vi "Transfer Function.vi"(3 "dt":dbl=1.0 format="%0.2f", 4 "Response Signal":dbl[](array[numeric]), 5 "Stimulus Signal":dbl[](array[numeric])) -> (0 "df":dbl format="%0.2f", 1 "Frequency Response Phase (radians)":dbl[](array[numeric]), 2 "Frequency Response Mag (gain)":dbl[](array[numeric]))   [LabVIEW 2020, in "NI_AALPro.lvlib"]
doc: "Computes the single-sided transfer function, also known as the frequency response, from the time-domain <B>Stimulus Signal</B> and <B>Response Signal</B> from a network under test."
uses:
  NI_AALPro.lvlib
  Real FFT.vi
panel:
  # "Transfer Function"
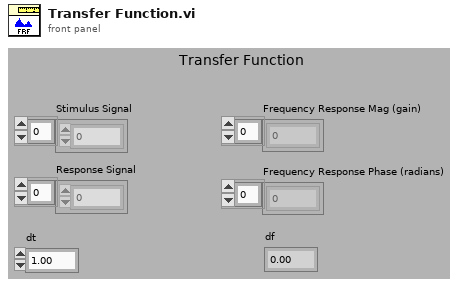
[diagram p1: front panel]
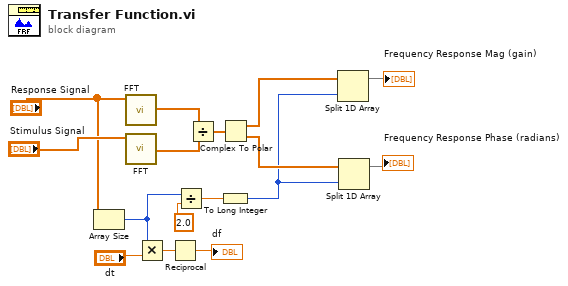
[diagram p0: block diagram]
diagram:
  n1 = Array Size(array="Response Signal") -> (size(s)=w5:i32)
  n2 = call-poly "FFT.vi"("X"="Response Signal") -> ("FFT {X}"=w3:cdb[])  [unwired: 9 in, 1 out]
  n3 = call-poly "FFT.vi"("X"="Stimulus Signal") -> ("FFT {X}"=w2:cdb[])  [unwired: 9 in, 1 out]
  n4 = Multiply(x=w5, y="dt") -> (x*y=w13:dbl)
  n5 = Reciprocal(x=w13) -> (1/x=→"df":dbl)
  n6 = Divide(x=w5, y=2.0) -> (x/y=w14:dbl)
  n7 = Divide(x=w3, y=w2) -> (x/y=w1:cdb[])
  n8 = To Long Integer(number=w14) -> (32bit integer=w4:i32)
  n9 = Complex To Polar(r * e^(i*theta)=w1) -> (r=w8:dbl[], theta=w15:dbl[])
  n10 = Split 1D Array(array=w8, index=w4) -> (first subarray=→"Frequency Response Mag (gain)":dbl[])  [unwired: 1 out]
  n11 = Split 1D Array(array=w15, index=w4) -> (first subarray=→"Frequency Response Phase (radians)":dbl[])  [unwired: 1 out]
